vi "Формирование кластера параметров мишени (SubVI).vi"(0 "Знак перемещения Dx":i8, 1 "выстрел X мишени":u16, 2 "выстрел Y мишени":u16, 7 "error in (no error)":errorcluster, 9 "Параметры Мишени":T1, 12 "номер мишени (id)":u8) -> (23 "Кластер параметров мишени":T2, 27 "error out":errorcluster)   [LabVIEW 2015]
doc: "Сворачивание всех параметров мишени в кластер"
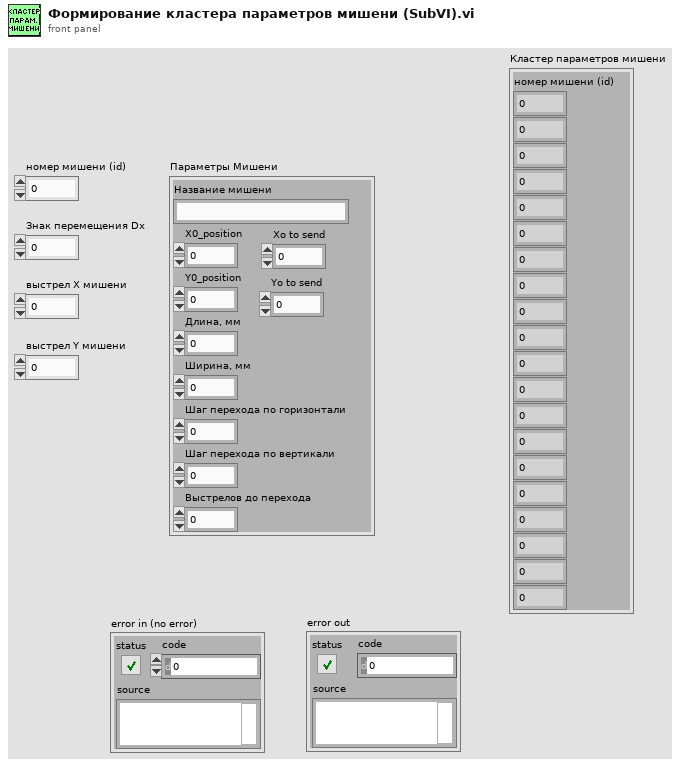
[diagram p1: front panel]
types:
  T1 = cluster{"Название мишени":string, "Х0_position":u16, "Y0_position":u16, "Длина, мм":u16, "Ширина, мм":u16, "Шаг перехода по горизонтали":dbl, "Шаг перехода по вертикали":dbl, "Выстрелов до перехода":u16, "Xo to send ":u16, "Yo to send":u16}
  T2 = cluster{"номер мишени (id)":u8, u8, u8, u8, u8, u8, u8, u8, u8, u8, u8, u8, u8, u8, u8, u8, u8, u8, u8, u8}
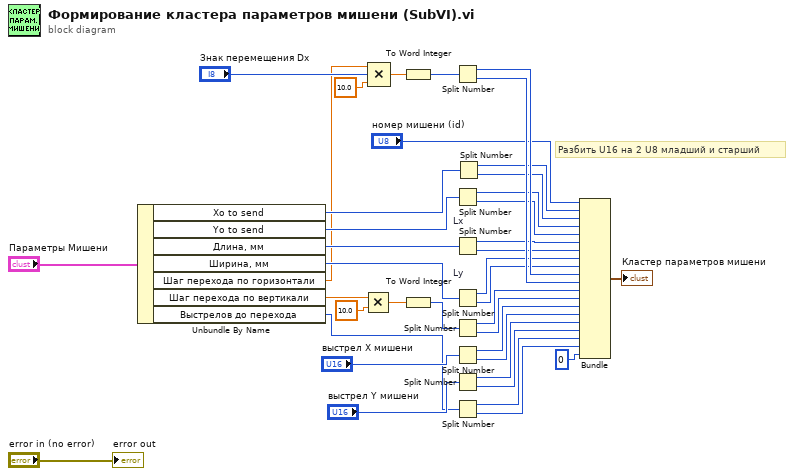
[diagram p0: block diagram]
diagram:
  # "Разбить U16 на 2 U8 младший и старший"
  n1 = Unbundle By Name("Параметры Мишени") -> ("Xo to send"=w7:u16, "Yo to send"=w6:u16, "Длина, мм"=w5:u16, "Ширина, мм"=w4:u16, "Шаг перехода по горизонтали"=w3:dbl, "Шаг перехода по вертикали"=w2:dbl, "Выстрелов до перехода"=w1:u16)
  n2 = Multiply(x=w2, y=10.0) -> (x*y=w13:dbl)
  n3 = Compound Arithmetic op=MULTIPLY(w3, "Знак перемещения Dx", 10.0 ("y")) -> (w17:dbl)
  n4 = To Word Integer(number=w17) -> (16bit integer=w15:i16)
  n5 = To Word Integer(number=w13) -> (16bit integer=w11:i16)
  n6 = Split Number(x=w15) -> (hi(x)=w29:u8, lo(x)=w30:u8)
  n7 = Split Number(x=w6) -> (hi(x)=w23:u8, lo(x)=w24:u8)
  n8 = Split Number "Lx"(x=w5) -> (hi(x)=w25:u8, lo(x)=w26:u8)
  n9 = Split Number "Ly"(x=w4) -> (hi(x)=w27:u8, lo(x)=w28:u8)
  n10 = Split Number(x=w11) -> (hi(x)=w31:u8, lo(x)=w32:u8)
  n11 = Split Number(x="выстрел X мишени") -> (hi(x)=w33:u8, lo(x)=w34:u8)
  n12 = Split Number(x="выстрел Y мишени") -> (hi(x)=w35:u8, lo(x)=w36:u8)
  n13 = Split Number(x=w1) -> (hi(x)=w37:u8, lo(x)=w38:u8)
  n14 = Split Number(x=w7) -> (hi(x)=w21:u8, lo(x)=w22:u8)
  n15 = Bundle("номер мишени (id)"="номер мишени (id)", w21, w22, w23, w24, w25, w26, w27, w28, w29, w30, w31, w32, w33, w34, w35, w36, w37, w38, u8 0) -> (→"Кластер параметров мишени":T2)  [unwired: 1 in]
  "error out" <- "error in (no error)"
